vi "Configure Sweep Trigger.vi"(0 "VISA resource name":refnum<visa-resource-name>, 1 "Point Trigger (1: Immediate)":u16(ring)=1 items=["Bus", "Immediate", "External", "Key", "Timer", "Manual", "Internal"], 2 "Enable Continuous Sweep (T:Enable)":bool=TRUE, 5 "Sweep Trigger (1: Immediate)":u16(ring)=1 items=["Bus", "Immediate", "External", "Key", "Timer", "Manual", "Internal"], 7 "Trigger Out Polarity (0: Positive)":u16(ring) items=["Positive", "Negative"], 9 "Trigger In Polarity (0: Positive)":u16(ring) items=["Positive", "Negative"], 11 "error in (no error)":errorcluster, 12 "Timer Trigger Period (1 ms)":dbl=0.001) -> (4 "VISA resource name out":refnum<visa-resource-name>, 15 "error out":errorcluster)   [LabVIEW 2018, in "Agilent PSG MXG Series.lvlib"]
doc: "Configures the trigger for list or step sweep."
uses:
  Agilent PSG MXG Series.lvlib
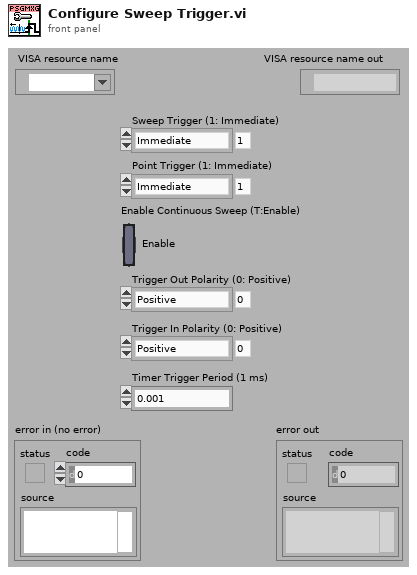
[diagram p1: front panel]
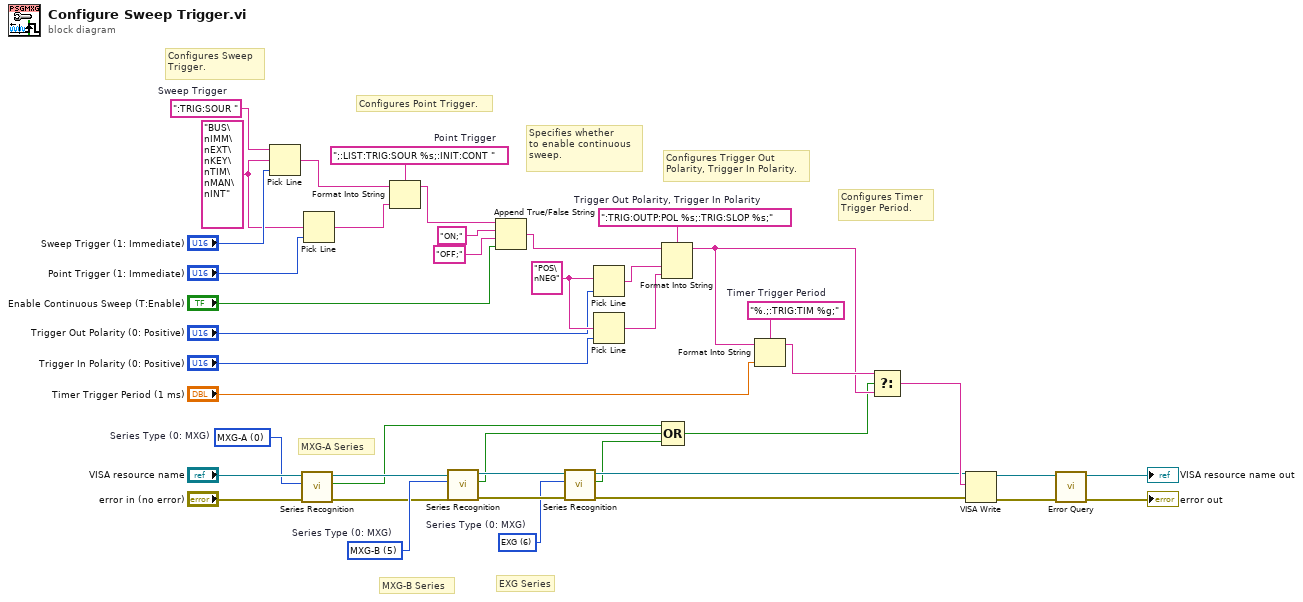
[diagram p0: block diagram]
diagram:
  w5 = u16 6 items=["MXG-A", "PSG", "PSG-A", "PSG-C", "PSG-D", "MXG-B", "EXG"]  # Series Type (0: MXG)
  w12 = u16 5 items=["MXG-A", "PSG", "PSG-A", "PSG-C", "PSG-D", "MXG-B", "EXG"]  # Series Type (0: MXG)
  w13 = u16 0 items=["MXG-A", "PSG", "PSG-A", "PSG-C", "PSG-D", "MXG-B", "EXG"]  # Series Type (0: MXG)
  w25 = "%.;:TRIG:TIM %g;"  # Timer Trigger Period
  w29 = "POS\nNEG" ("multi-line string")
  w31 = ":TRIG:OUTP:POL %s;:TRIG:SLOP %s;"  # Trigger Out Polarity, Trigger In Polarity
  w38 = ";:LIST:TRIG:SOUR %s;:INIT:CONT "  # Point Trigger
  w40 = "BUS\nIMM\nEXT\nKEY\nTIM\nMAN\nINT" ("multi-line string")
  w42 = ":TRIG:SOUR "  # Sweep Trigger
  # "EXG Series"
  # "MXG-B Series"
  # "Configures Timer\nTrigger Period."
  # "Configures Trigger Out\nPolarity, Trigger In Polarity."
  # "Specifies whether\nto enable continuous\nsweep."
  # "Configures Point Trigger."
  # "Configures Sweep\nTrigger."
  # "MXG-A Series"
  n1 = Pick Line(string ("")=w42, multi-line string=w40, line index="Sweep Trigger (1: Immediate)") -> (output string=w37:string)
  n2 = call "Series Recognition.vi"("error in (no error)"="error in (no error)", "Series Type (0: MXG)"=w13, "VISA resource name"="VISA resource name") -> ("error out"=w10:errorcluster, "Is Series Correct"=w4:bool, "VISA resource name out"=w11:refnum<visa-resource-name>)  [unwired: 6 out]
  n3 = Pick Line(multi-line string=w40, line index="Point Trigger (1: Immediate)") -> (output string=w36:string)  [unwired: 1 out]
  n4 = Format Into String(format string=w38, initial string=w37, w36) -> (resulting string=w35:string)  [unwired: 1 in, 1 out]
  n5 = call "Series Recognition.vi"("error in (no error)"=w10, "Series Type (0: MXG)"=w12, "VISA resource name"=w11) -> ("error out"=w7:errorcluster, "Is Series Correct"=w3:bool, "VISA resource name out"=w9:refnum<visa-resource-name>)  [unwired: 6 out]
  n6 = Append True/False String(1:"Enable Continuous Sweep (T:Enable)", 2:"OFF;" ("false string"), 3:"ON;" ("true string"), 4:w35) -> (0:w32:string)
  n7 = call "Series Recognition.vi"("error in (no error)"=w7, "Series Type (0: MXG)"=w5, "VISA resource name"=w9) -> ("error out"=w6:errorcluster, "Is Series Correct"=w2:bool, "VISA resource name out"=w8:refnum<visa-resource-name>)  [unwired: 6 out]
  n8 = Pick Line(multi-line string=w29, line index="Trigger Out Polarity (0: Positive)") -> (output string=w30:string)  [unwired: 1 out]
  n9 = Pick Line(multi-line string=w29, line index="Trigger In Polarity (0: Positive)") -> (output string=w26:string)  [unwired: 1 out]
  n10 = Format Into String(format string=w31, initial string=w32, w30, w26) -> (resulting string=w22:string)  [unwired: 1 in, 1 out]
  n11 = Compound Arithmetic op=OR(w4, w3, w2) -> (w1:bool)
  n12 = Format Into String(format string=w25, initial string=w22, "Timer Trigger Period (1 ms)") -> (resulting string=w23:string)  [unwired: 1 in, 1 out]
  n13 = Select(t=w23, s=w1, f=w22) -> (s? t:f=w21:string)
  n14 = VISA Write(VISA resource name=w8, write buffer=w21, error in (no error)=w6) -> (VISA resource name out=w20:refnum<visa-resource-name>, error out=w19:errorcluster)  [unwired: 1 out]
  n15 = call "Error Query.vi"("error in (no error)"=w19, "VISA resource name"=w20) -> ("error out"=→"error out":errorcluster, "VISA resource name out"=→"VISA resource name out":refnum<visa-resource-name>)  [unwired: 8 out]
